vi "GetProperties.vi"(8 "error in":errorcluster, 11 "Tab in":refnum<class "Tab.lvclass">) -> (0 "error out":errorcluster, 3 "Tab out":refnum<class "Tab.lvclass">)   [LabVIEW 2014, in "Raspberry Pi Compatible Compiler for LabVIEW.lvlib" / "Tab.lvclass"]
uses:
  Tab.lvclass
  Tab.lvclass/Tab.ctl
  PageSelector/PageSelector.lvclass
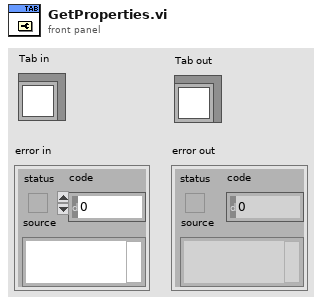
[diagram p1: front panel]
types:
  T1 = typedef "LVForegroundBackgroundColorsTypeDef.ctl" = cluster{"FG Color":u32, "BG Color":u32}
  T2 = typedef "LVBoundsTypeDef.ctl" = cluster{"Width":u32, "Height":u32}
  T3 = enum32{"Text Only", "Image Only", "Text - Image", "Image - Text"}
  T4 = enum32{"Size Tabs To Contents", "Size All Tabs to Largest Tab", "Fixed Tab Size"}
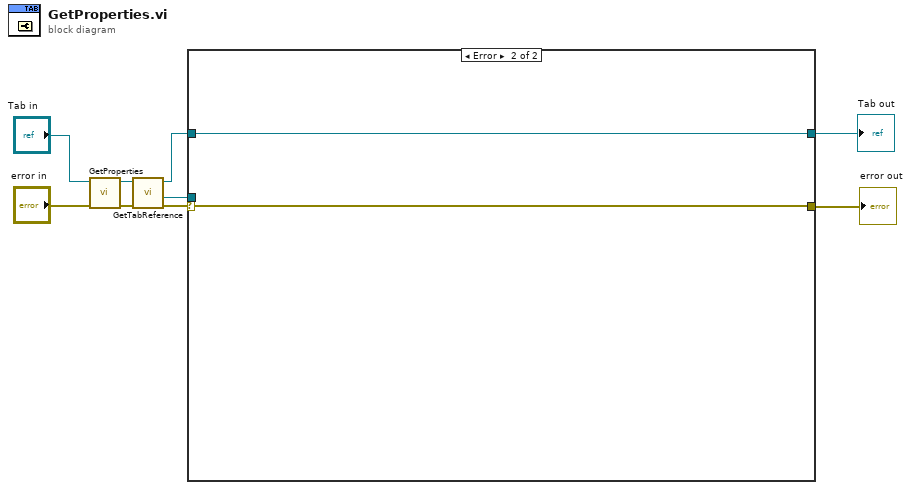
[diagram p0: block diagram]
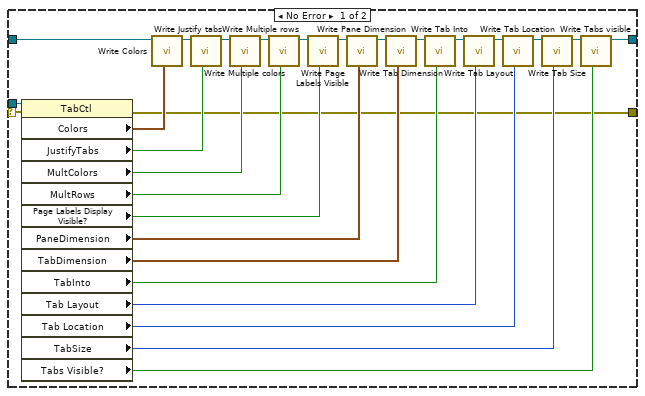
[diagram p2: hidden frame]
diagram:
  n1 = call-parent "GetProperties.vi"("error in"="error in", "PageSelector in"="Tab in") -> ("error out"=w6:errorcluster, "PageSelector out"=w7:refnum<class "Tab.lvclass">)  [unwired: 8 in]
  n2 = call "GetTabReference.vi"("error in"=w6, "Tab in"=w7) -> ("error out"=w5:errorcluster, "tab reference"=w4:refnum<vi>, "Tab out"=w3:refnum<class "Tab.lvclass">)  [unwired: 7 in]
  n3 = case shown="Error" w5 {
    selector: w5 -> [w36 w38]
    tunnel: w4 -> [w37 _]
    tunnel: w3 -> [w12 w39]
    tunnel: [w11 w39] -> w2
    tunnel: [w10 w38] -> w1
    frame No Error {
      n4 = property class="TabCtl"(reference=w37, error in=w36) -> (error out=w10:errorcluster, "Colors"=w24:T1, "JustifyTabs"=w23:bool, "MultColors"=w22:bool, "MultRows"=w21:bool, "Page Labels Display Visible?"=w20:bool, "PaneDimension"=w19:T2, "TabDimension"=w18:T2, "TabInto"=w17:bool, "Tab Layout"=w16:T3, "Tab Location"=w15:enum32{"Top", "Bottom", "Left", "Right"}, "TabSize"=w14:T4, "Tabs Visible?"=w13:bool)  [unwired: 1 out]
      n5 = call "Write Colors.vi"("Colors"=w24, "Tab in"=w12) -> ("Tab out"=w35:refnum<class "Tab.lvclass">)  [unwired: 7 in]
      n6 = call "Write Justify tabs.vi"("Justify tabs"=w23, "Tab in"=w35) -> ("Tab out"=w34:refnum<class "Tab.lvclass">)  [unwired: 7 in]
      n7 = call "Write Multiple colors.vi"("Multiple colors"=w22, "Tab in"=w34) -> ("Tab out"=w33:refnum<class "Tab.lvclass">)  [unwired: 7 in]
      n8 = call "Write Multiple rows.vi"("Multiple rows"=w21, "Tab in"=w33) -> ("Tab out"=w32:refnum<class "Tab.lvclass">)  [unwired: 7 in]
      n9 = call "Write Page Labels Visible.vi"("Page Labels Visible"=w20, "Tab in"=w32) -> ("Tab out"=w31:refnum<class "Tab.lvclass">)  [unwired: 7 in]
      n10 = call "Write Pane Dimension.vi"("Pane Dimension"=w19, "Tab in"=w31) -> ("Tab out"=w30:refnum<class "Tab.lvclass">)  [unwired: 7 in]
      n11 = call "Write Tab Dimension.vi"("Tab Dimension"=w18, "Tab in"=w30) -> ("Tab out"=w29:refnum<class "Tab.lvclass">)  [unwired: 7 in]
      n12 = call "Write Tab Into.vi"("Tab Into"=w17, "Tab in"=w29) -> ("Tab out"=w28:refnum<class "Tab.lvclass">)  [unwired: 7 in]
      n13 = call "Write Tab Layout.vi"("Tab Layout"=w16, "Tab in"=w28) -> ("Tab out"=w27:refnum<class "Tab.lvclass">)  [unwired: 7 in]
      n14 = call "Write Tab Location.vi"("Tab Location"=w15, "Tab in"=w27) -> ("Tab out"=w26:refnum<class "Tab.lvclass">)  [unwired: 7 in]
      n15 = call "Write Tab Size.vi"("Tab Size"=w14, "Tab in"=w26) -> ("Tab out"=w25:refnum<class "Tab.lvclass">)  [unwired: 7 in]
      n16 = call "Write Tabs visible.vi"("Tabs visible"=w13, "Tab in"=w25) -> ("Tab out"=w11:refnum<class "Tab.lvclass">)  [unwired: 7 in]
    }
    frame Error {
    }
  }
  "error out" <- w1
  "Tab out" <- w2
